vi "JSON to LVObject - Warning Input - Returns Specified Object.vi"() -> ()   [LabVIEW 2017, in "Generic Object Serializer Tests.lvlib"]
uses:
  Generic Object Serializer Tests.lvlib
  Weather Forecast/Weather Forecast.lvclass
  Generic Object Serializer/Generic Object Serializer.lvclass
  <vilib>/Utility/error.llb/Error Cluster From Error Code.vi
  <vilib>/addons/_JKI Toolkits/Caraya/classes/Assert/Assert Equal Value and Type_Variant.vi
  <vilib>/ErrorRing/Error Ring.xnode
  <vilib>/addons/_JKI Toolkits/Caraya/classes/Test/Test.lvclass
  <vilib>/addons/_JKI Toolkits/Caraya/classes/Assert/Assert.lvclass
panel:
  out "error out":errorcluster
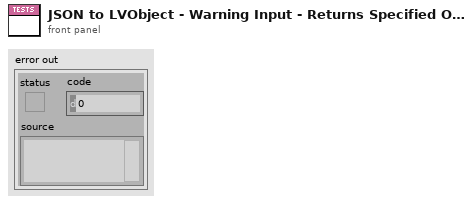
[diagram p1: front panel]
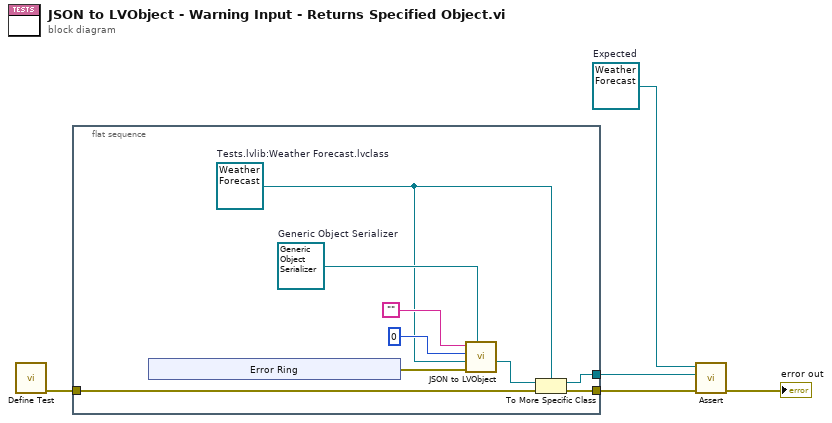
[diagram p0: block diagram]
diagram:
  w1 = refnum<class "Weather Forecast.lvclass"> refnum  # Expected
  n1 = call <vilib>:"Define Test.vi"() -> ("error out"=w4:errorcluster)  [unwired: 11 in]
  n2 = flat-sequence {
    tunnel: w4 -> [w13]
    tunnel: [w9] -> w3
    tunnel: [w7] -> w2
    frame #0 {
      w6 = refnum<class "Weather Forecast.lvclass"> refnum  # Tests.lvlib:Weather Forecast.lvclass
      w14 = refnum<class "Generic Object Serializer.lvclass"> refnum  # Generic Object Serializer
      n3 = xnode "Error Ring"() -> ("error out"=w12:errorcluster)
      n4 = call-dynamic "JSON to LVObject.vi"("LVClass Serializer"=w14, "error in (no error)"=w12, "Object Type"=w6, "Offset"=0, "JSON"="") -> ("Object"=w8:refnum<class>)  [unwired: 5 in, 1 out]
      n5 = To More Specific Class(target class=w6, reference=w8, error in=w13) -> (specific class reference=w7:refnum<class "Weather Forecast.lvclass">, error out=w9:errorcluster)
    }
  }
  n6 = call-poly <vilib>:"Assert.vi"("error in (no error)"=w3, "Y"=w2, "X"=w1) -> ("error out"=→"error out":errorcluster)  [unwired: 8 in]
